vi "Append Properties To Edit Context Menu.vi"(9 "State":T1, 11 "Menu in":refnum<k9>) -> ()   [LabVIEW 2020, in "Waveform (G3).xctl"]
uses:
  Waveform (G3).xctl
  State.ctl
  Utility VIs/Controls/KRing/KRing.xctl
  Tone (G3)/Tone (G3).xctl
  Noise (G3)/Noise (G3).xctl
  Noise (G3)/Noise (G3) - Persistent.ctl
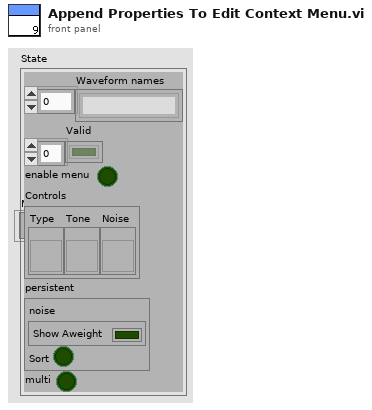
[diagram p1: front panel]
types:
  T1 = typedef "Waveform (G3).xctl/State.ctl" = cluster{"Waveform names":string[], "Valid":bool[], "enable menu":bool, "Controls":cluster{"Type ":refnum<vi>, "Tone ":refnum<vi>, "Noise":refnum<vi>}, "persistent":cluster{"noise":T2, "Sort":bool}, "multi":bool}
  T2 = typedef "Noise (G3).xctl/Noise (G3) - Persistent.ctl" = cluster{"Show Aweight":bool}
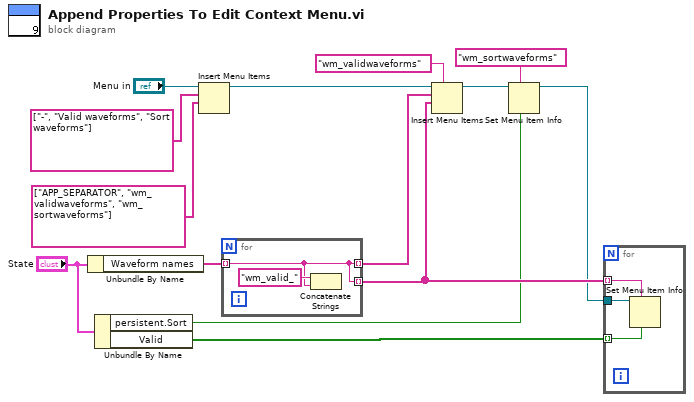
[diagram p0: block diagram]
diagram:
  n1 = Unbundle By Name("State") -> ("Waveform names"=w9:string[])
  n2 = Unbundle By Name("State") -> ("persistent.Sort"=w1:bool, "Valid"=w5:bool[])
  n3 = Insert Menu Items(7:string[] ["APP_SEPARATOR", "wm_validwaveforms", "wm_sortwaveforms"] ("item names"), 8:string[] ["-", "Valid waveforms", "Sort waveforms"] ("item names"), 9:"Menu in") -> (3:w13:refnum<k9>)  [unwired: 3 in, 2 out]
  n4 = for {
    tunnel: w9 -> [w15] mode=indexing
    tunnel: [w15] -> w8 mode=indexing
    tunnel: [w15] -> w7 mode=indexing
    n5 = Concatenate Strings("wm_valid_" ("string"), w15) -> ()  [unwired: 1 out]
  }
  n6 = Insert Menu Items(5:"wm_validwaveforms", 7:w7, 8:w8, 9:w13) -> (3:w4:refnum<k9>)  [unwired: 2 in, 2 out]
  n7 = Set Menu Item Info(6:w1, 7:"wm_sortwaveforms", 11:w4) -> (3:w3:refnum<k9>)  [unwired: 4 in, 1 out]
  n8 = for {
    tunnel: w3 -> [w19]
    tunnel: w7 -> [w18] mode=indexing
    tunnel: w5 -> [w17] mode=indexing
    n9 = Set Menu Item Info(6:w17, 7:w18, 11:w19) -> ()  [unwired: 4 in, 2 out]
  }
